vi "N03_Decision.vi"() -> ()   [LabVIEW 2023]
panel:
  out "Case Output":dbl
  in  "Boolean":bool
  out "Select Output":dbl
  in  "False Numeric":dbl
  in  "True Numeric":dbl
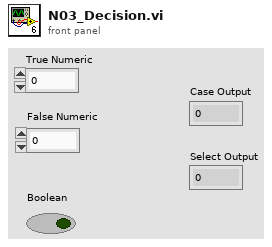
[diagram p1: front panel]
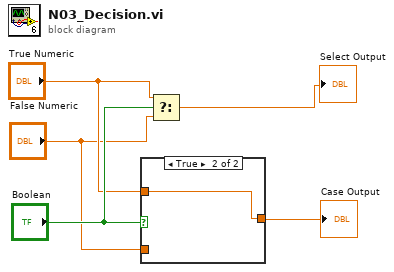
[diagram p0: block diagram]
diagram:
  n1 = case shown="True" "Boolean" {
    tunnel: "True Numeric" -> [_ w7]
    tunnel: "False Numeric" -> [w6 _]
    tunnel: [w6 w7] -> w1
    frame False {
    }
    frame True {
    }
  }
  "Case Output" <- w1
  n2 = Select(t="True Numeric", s="Boolean", f="False Numeric") -> (s? t:f=→"Select Output":dbl)
